vi "Test EMD.vi"() -> ()   [LabVIEW 2013]
uses:
  <vilib>/Waveform/WDTOps.llb/WDT Get Waveform Subset DBL.vi
  <vilib>/measure/maresamp.llb/Resample Waveform (single shot).vi
  <vilib>/Waveform/WDTFileIO.llb/ Write Waveforms to File (1D).vi
  <vilib>/Waveform/WDTFileIO.llb/Export Waveforms To Spreadsheet File (1D).vi
  Empirical Mode Decomposition.lvlib
  <vilib>/measure/NI_MAPro.lvlib
panel:
  in  "HHT":bool
  in  "Filter":bool
  in  "Upsample":bool
  in  "start samples/time":dbl format="%#.6g"
  in  "duration (s)":dbl=0.0001
  out "Signal":waveform(dbl)(graph)
  out "Hilbert Spectrum":dbl[][](graph)
  out "IMF":waveform(dbl)(graph)
  in  "Image Base Path":path
  out "dt":dbl
  out "df":dbl
  in  "Save":bool
  in  "Record Index":i32
  in  "Channel Index":i32
  in  "IMF Tolerance":dbl=0.2 format="%#_13g"
  out "error out":errorcluster
  out "Records read":i32
  in  "File path":path
  # ".296+.003"
  # ".162+.004"
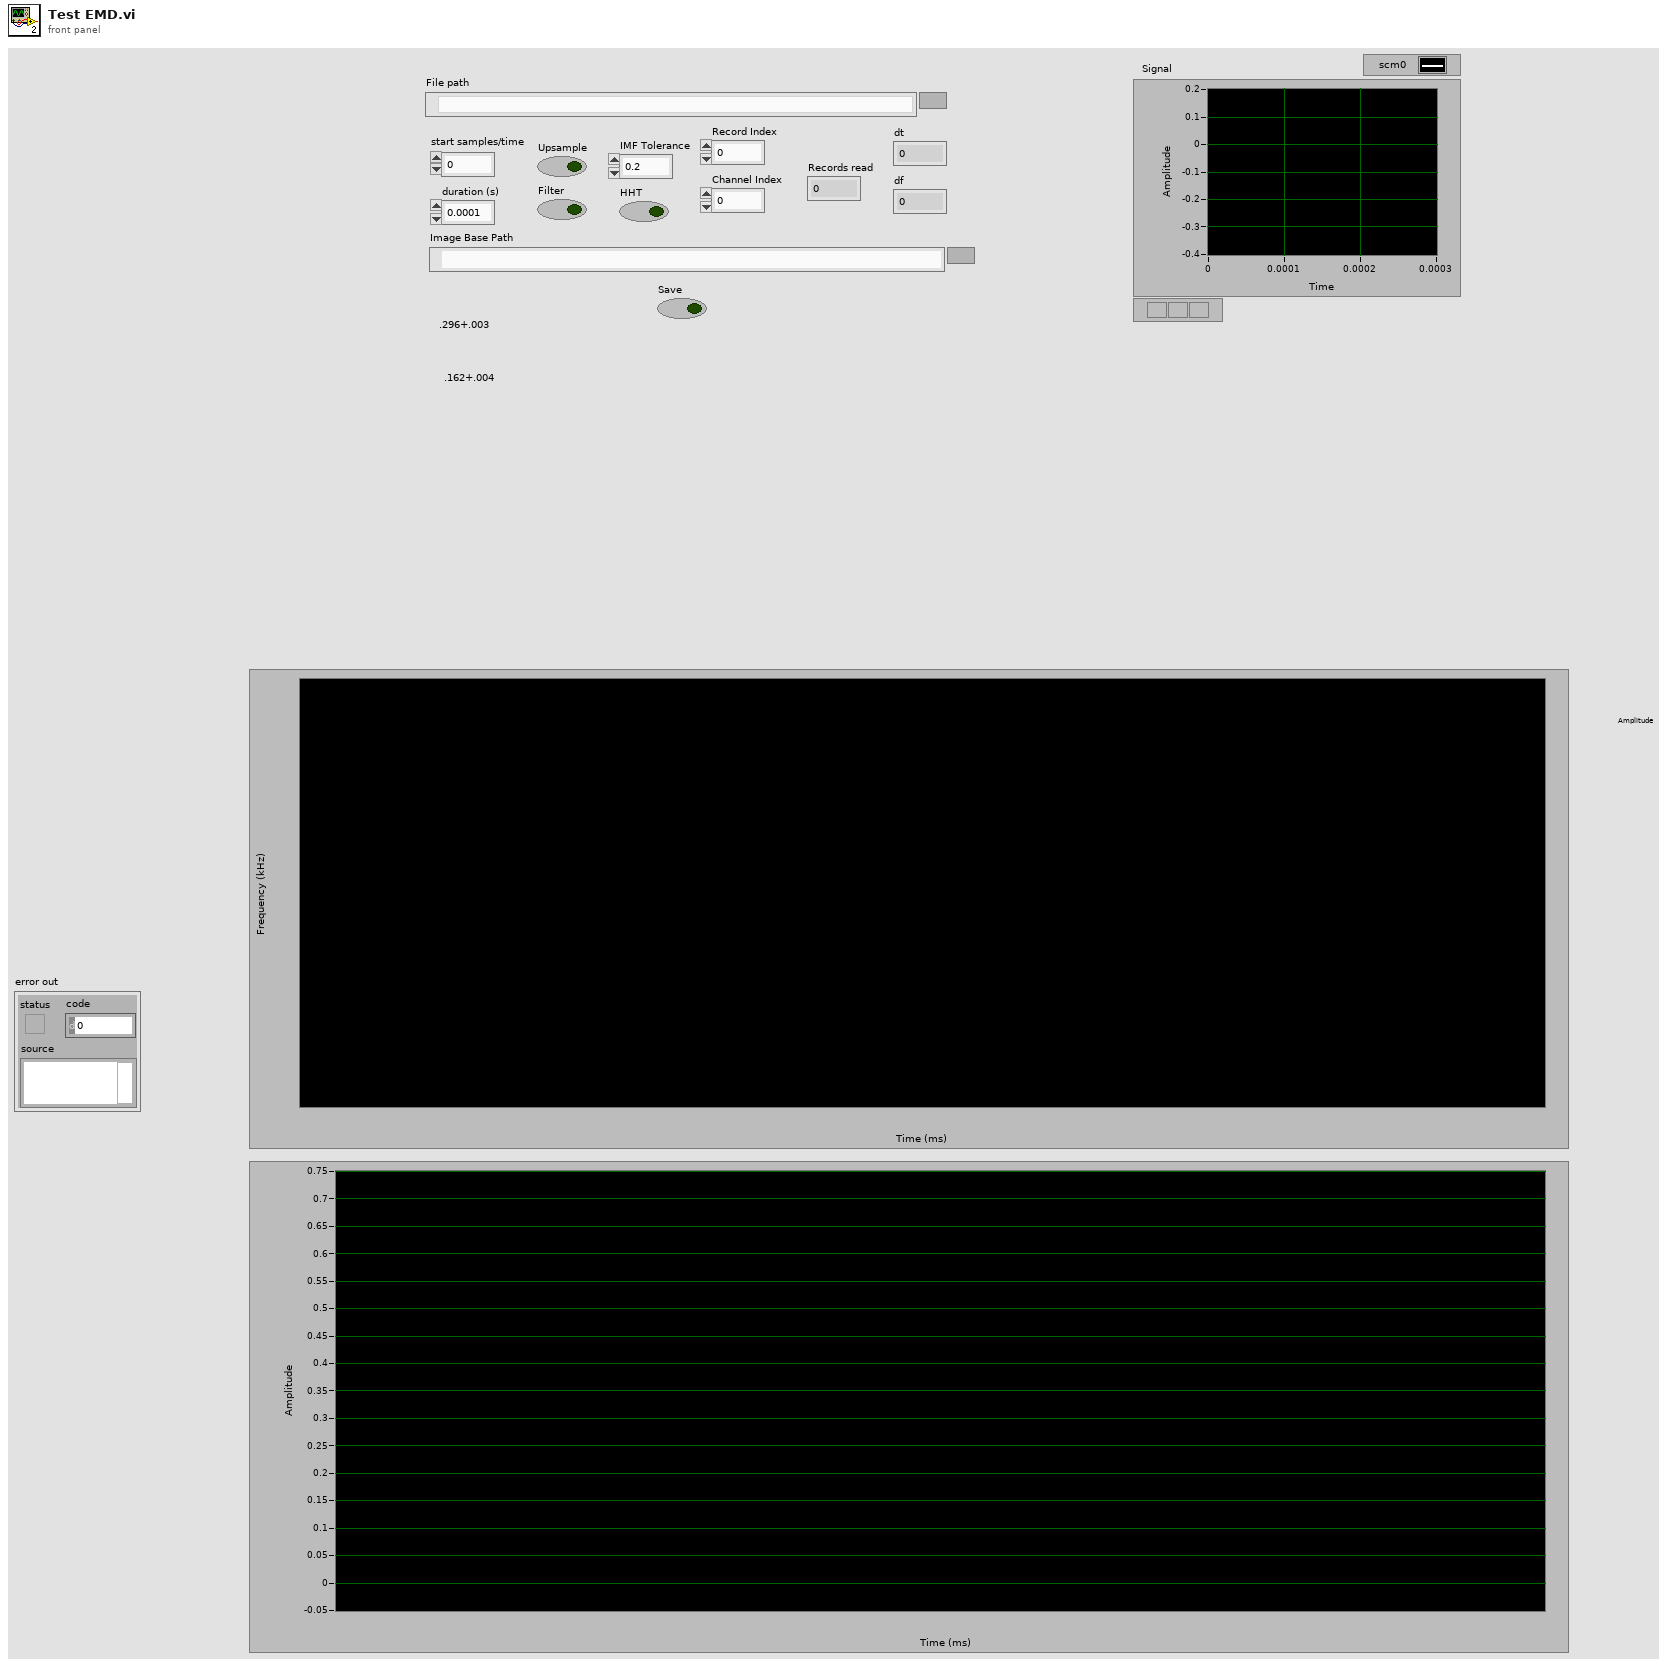
[diagram p1: front panel]
types:
  T1 = typedef "imagedata.ctl" = cluster{"image type":i32, "image depth":i32, "image":u8[], "mask":u8[], "colors":u32[], "Rectangle":cluster{"left":i16, "top":i16, "right":i16, "bottom":i16}}
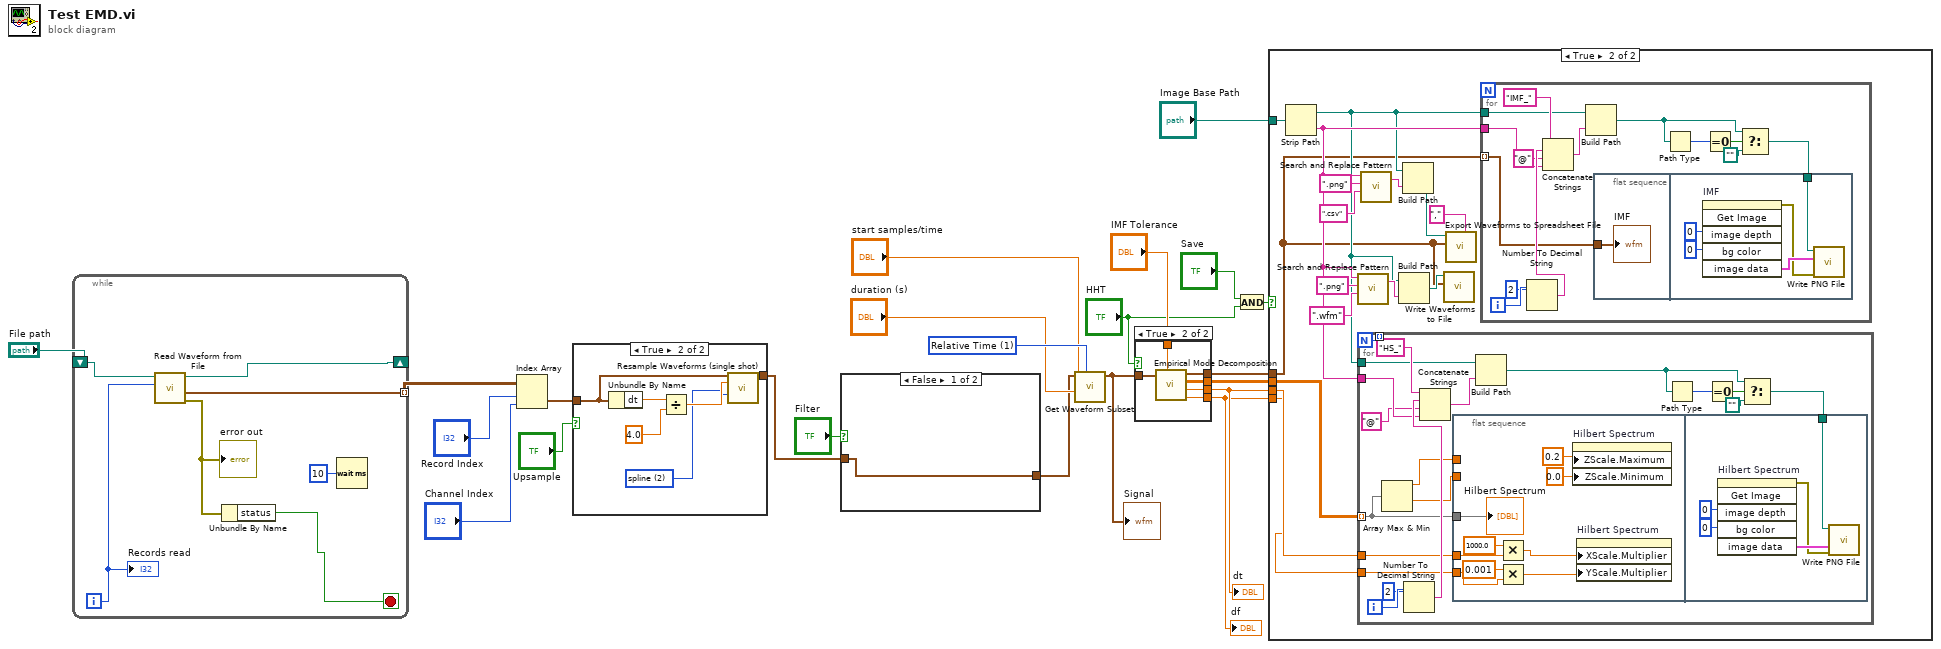
[diagram p0: block diagram]
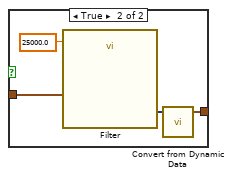
[diagram p3: hidden frame]
diagram:
  w19 = u16 1 items=["Samples", "Relative Time"] ("start/duration format")
  n1 = while {
    tunnel: [w25] -> w22 mode=indexing
    shift-right: [w24] -> _
    shift-left: "File path" -> [w23]
    i -> [w28]
    stop <- w27 stop-if-true
    n2 = call <vilib>:"Read Waveform from File.vi"("offset (records:0)"=w28, "file path (dialog if empty)"=w23) -> ("error out"=w29:errorcluster, "all waveforms in record"=w25:waveform(dbl)[], "new file path (Not A Path if cancelled)"=w24:path)  [unwired: 4 in, 1 out]
    "error out" <- w29
    n3 = Unbundle By Name(w29) -> ("status"=w27:bool)
    n4 = Wait (ms)(milliseconds to wait=u32 10) -> ()  [unwired: 1 out]
    "Records read" <- w28
  }
  n5 = Index Array(array=w22, index (row)="Record Index", index (col)="Channel Index") -> (element=w9:waveform(dbl))
  n6 = case shown="True" "Upsample" {
    tunnel: w9 -> [w30 w32]
    tunnel: [w30 w31] -> w6
    frame False {
    }
    frame True {
      w33 = u16 2 items=["coerce", "linear", "spline", "FIR filter"] ("interpolation mode")
      n7 = Unbundle By Name(w32) -> ("dt"=w36:dbl)
      n8 = Divide(x=w36, y=4.0) -> (x/y=w34:dbl)
      n9 = call-poly <vilib>:"Resample Waveforms (single shot).vi"("waveform in"=w32, "dt"=w34, "interpolation mode"=w33) -> ("resampled waveform out"=w31:waveform(dbl))  [unwired: 9 in, 3 out]
    }
  }
  n10 = case shown="False" "Filter" {
    tunnel: w6 -> [w37 w40]
    tunnel: [w37 w38] -> w4
    frame False {
    }
    frame True {
      n11 = call "Filter"("Lower Cut-Off"=25000.0, "Signal"=w40) -> ("Filtered Signal"=w39:dynamicdata)  [unwired: 8 in, 1 out]
      n12 = call "Convert from Dynamic Data"("Dynamic Data Type"=w39) -> ("Waveform"=w38:waveform(dbl))  [unwired: 3 in]
    }
  }
  n13 = call-poly <vilib>:"Get Waveform Subset.vi"("start/duration format"=w19, "duration"="duration (s)", "start samples/time"="start samples/time", "waveform in"=w4) -> ("waveform out"=w10:waveform(dbl))  [unwired: 2 in, 3 out]
  "Signal" <- w10
  n14 = case shown="True" "HHT" {
    tunnel: "IMF Tolerance" -> [_ w47]
    tunnel: [_ w46] -> w15
    tunnel: [_ w45] -> w14
    tunnel: [_ w44] -> w12
    tunnel: [_ w43] -> w11
    tunnel: w10 -> [_ w42]
    frame False {
    }
    frame True {
      n15 = call "Empirical Mode Decomposition.vi"("IMF Tolerance"=w47, "Waveform"=w42) -> ("df"=w43:dbl, "dt"=w44:dbl, "Hilbert Spectra"=w45:dbl[][][], "IMF Array"=w46:waveform(dbl)[])  [unwired: 6 in]
    }
  }
  "df" <- w11
  "dt" <- w12
  n16 = And(x="Save", y="HHT") -> (x .and. y?=w3:bool)
  n17 = case shown="True" w3 {
    tunnel: w15 -> [_ w48]
    tunnel: w14 -> [_ w60]
    tunnel: "Image Base Path" -> [_ w63]
    tunnel: w12 -> [_ w62]
    tunnel: w11 -> [_ w61]
    frame False {
    }
    frame True {
      n18 = Strip Path(path=w63) -> (stripped path=w50:path, name=w52:string)
      n19 = call <vilib>:"Search and Replace Pattern.vi"("string"=w52, "regular expression (\"\")"=".png" ("regular expression (\"\")"), "replace string (\"\")"=".wfm" ("replace string (\"\")")) -> ("result string"=w51:string)  [unwired: 2 in, 1 out]
      n20 = for {
        N -> [w64]
        tunnel: w50 -> [w73]
        tunnel: w52 -> [w74]
        tunnel: w62 -> [w70]
        tunnel: w61 -> [w69]
        tunnel: w60 -> [w68] mode=indexing
        tunnel: [w64] -> _ mode=indexing
        i -> [w77]
        n21 = Array Max & Min(array=w68) -> (max value=w67:dbl, min value=w66:dbl)  [unwired: 2 out]
        n22 = Number To Decimal String(number=w77, width (-)=i16 2) -> (decimal integer string=w76:string)
        n23 = Concatenate Strings("HS_" ("search string/char (-)"), w76, "@" ("string"), w74) -> (w72:string)
        n24 = flat-sequence {
          tunnel: w70 -> [w88]
          tunnel: w69 -> [w84]
          tunnel: w68 -> [w91]
          tunnel: w67 -> [_]
          tunnel: w66 -> [_]
          tunnel: w80 -> [w93]
          frame #0 {
            n25 = Multiply(x=1000.0, y=w88) -> (x*y=w85:dbl)
            n26 = Multiply(x=0.001, y=w84) -> (x*y=w83:dbl)
            n27 = property on="Hilbert Spectrum" class="IntGraph (strict)"("ZScale.Maximum"=0.2 ("Z Scale.Range:Maximum"), "ZScale.Minimum"=0.0 ("Z Scale.Range:Minimum")) -> ()  [unwired: 2 in, 2 out]
            n28 = property on="Hilbert Spectrum" class="IntGraph (strict)"("XScale.Multiplier"=w85, "YScale.Multiplier"=w83) -> ()  [unwired: 2 in, 2 out]
            "Hilbert Spectrum" <- w91
          }
          frame #1 {
            n29 = invoke on="Hilbert Spectrum" class="IntGraph (strict)" method="Get Image"("image depth"=0 ("Image Depth"), "bg color"=u32 0 ("Background Color")) -> (error out=w92:errorcluster, "image data"=w94:T1)  [unwired: 4 in, 4 out]
            n30 = call <vilib>:"Write PNG File.vi"("error in (no error)"=w92, "image data"=w94, "path to PNG file"=w93) -> ()  [unwired: 7 in, 2 out]
          }
        }
        n31 = Build Path(base path=w73, name or relative path=w72) -> (appended path=w71:path)
        n32 = Path Type(1:w71) -> (0:w82:i16)
        n33 = Equal To 0?(x=w82) -> (x = 0?=w81:bool)
        n34 = Select(t=w71, s=w81, f=path "") -> (s? t:f=w80:path)
      }
      n35 = call <vilib>:"Search and Replace Pattern.vi"("string"=w52, "regular expression (\"\")"=".png" ("regular expression (\"\")"), "replace string (\"\")"=".csv" ("replace string (\"\")")) -> ("result string"=w57:string)  [unwired: 2 in, 1 out]
      n36 = Build Path(base path=w50, name or relative path=w51) -> (appended path=w49:path)
      n37 = Build Path(base path=w50, name or relative path=w57) -> (appended path=w55:path)
      n38 = call-poly <vilib>:"Write Waveforms to File.vi"("waveform array"=w48, "file path (dialog if empty)"=w49) -> ()  [unwired: 8 in, 2 out]
      n39 = call-poly <vilib>:"Export Waveforms to Spreadsheet File.vi"("delimiter (Tab)"=",", "waveforms"=w48, "file path (dialog if empty)"=w55) -> ()  [unwired: 7 in, 2 out]
      n40 = for {
        tunnel: w48 -> [w98] mode=indexing
        tunnel: w50 -> [w101]
        tunnel: w52 -> [w102]
        i -> [w105]
        n41 = Number To Decimal String(number=w105, width (-)=i16 2) -> (decimal integer string=w104:string)
        n42 = Concatenate Strings("IMF_" ("search string/char (-)"), w104, "@" ("string"), w102) -> (w100:string)
        n43 = Build Path(base path=w101, name or relative path=w100) -> (appended path=w99:path)
        n44 = flat-sequence {
          tunnel: w98 -> [w111]
          tunnel: w108 -> [w113]
          frame #0 {
            "IMF" <- w111
          }
          frame #1 {
            n45 = invoke on="IMF" class="WFGraph (strict)" method="Get Image"("image depth"=0 ("Image Depth"), "bg color"=u32 0 ("Background Color")) -> (error out=w112:errorcluster, "image data"=w114:T1)  [unwired: 4 in, 4 out]
            n46 = call <vilib>:"Write PNG File.vi"("error in (no error)"=w112, "image data"=w114, "path to PNG file"=w113) -> ()  [unwired: 7 in, 2 out]
          }
        }
        n47 = Path Type(1:w99) -> (0:w110:i16)
        n48 = Equal To 0?(x=w110) -> (x = 0?=w109:bool)
        n49 = Select(t=w99, s=w109, f=path "") -> (s? t:f=w108:path)
      }
    }
  }
